vi "snap test.vi"() -> ()   [LabVIEW 2013]
panel:
  out "Image Out":T1(plugin-control)
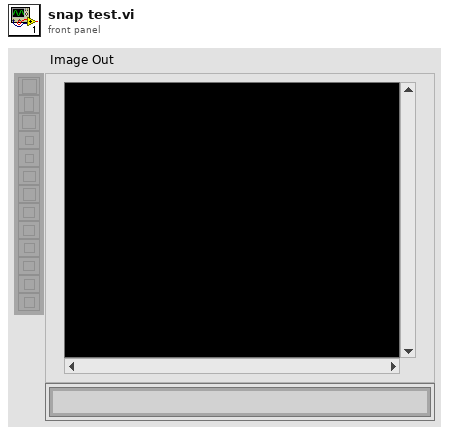
[diagram p1: front panel]
types:
  T1 = typedef "IMAQ Image.ctl" = refnum<image>
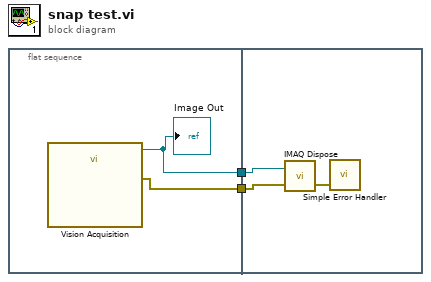
[diagram p0: block diagram]
diagram:
  n1 = flat-sequence {
    tunnel: [w4] -> w2
    tunnel: [w3] -> w1
    tunnel: w2 -> [w5]
    tunnel: w1 -> [w6]
    frame #0 {
      n2 = call "Vision Acquisition"() -> ("Image Out"=w3:T1, "error out"=w4:errorcluster)  [unwired: 26 in]
      "Image Out" <- w3
    }
    frame #1 {
      n3 = call "IMAQ Dispose"("Image"=w6, "error in (no error)"=w5) -> ("error out"=w7:errorcluster)  [unwired: 4 in]
      n4 = call <vilib>:"Simple Error Handler.vi"("error in (no error)"=w7) -> ()  [unwired: 4 in, 5 out]
    }
  }
